vi "popupHelpInfo.vi"(8 "error in":errorcluster, 11 "fileName":string) -> (0 "error out":errorcluster)   [LabVIEW 2010]
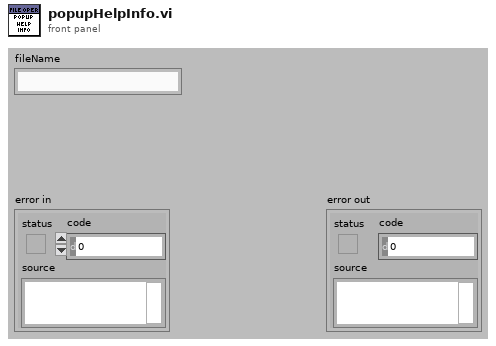
[diagram p1: front panel]
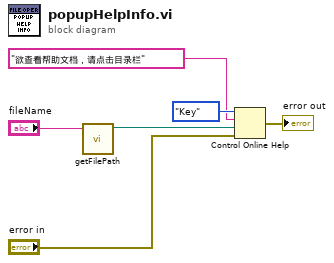
[diagram p0: block diagram]
diagram:
  n1 = call "getFilePath.vi"("fileName"="fileName") -> ("path"=w4:path)  [unwired: 10 in]
  n2 = Control Online Help(1:"error in", 2:w4, 3:"欲查看帮助文档，请点击目录栏" ("String to search for"), 4:enum16{"Contents", "Key", "Close"}."Key" ("Operation")) -> (0:→"error out":errorcluster)
